vi "Timeout Timer.vi"(1 "reset?(F)":bool, 2 "timeout(s)":dbl=5.0) -> (7 "timeout?":bool, 9 "time esliped?":dbl)   [LabVIEW 2017]
doc: "Reports whether the configured timeout has elapsed and returns the time since the timer was last reset."
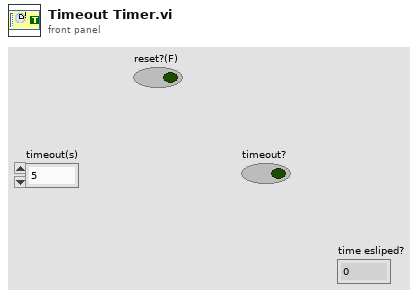
[diagram p1: front panel]
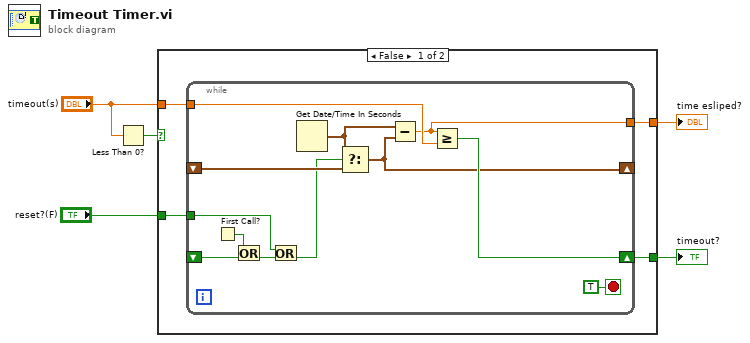
[diagram p0: block diagram]
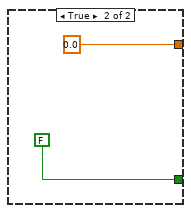
[diagram p2: hidden frame]
diagram:
  n1 = Less Than 0?(x="timeout(s)") -> (x < 0?=w4:bool)
  n2 = case shown="False" w4 {
    tunnel: "timeout(s)" -> [w9 _]
    tunnel: [w8 FALSE] -> w5
    tunnel: [w7 0.0] -> w2
    tunnel: "reset?(F)" -> [w6 _]
    frame False {
      n3 = while {
        shift-right: [w15] -> _
        shift-left: _ -> [w20]
        tunnel: w9 -> [w19]
        shift-right: [w18] -> w8
        shift-left: _ -> [w14]
        tunnel: [w17] -> w7
        tunnel: w6 -> [w10]
        stop <- TRUE stop-if-true
        n4 = First Call?() -> (First Call?: T/F=w12:bool)
        n5 = Or(x=w12, y=w14) -> (x .or. y?=w13:bool)
        n6 = Or(x=w10, y=w13) -> (x .or. y?=w11:bool)
        n7 = Get Date/Time In Seconds() -> (seconds since 1Jan1904=w16:timestamp)
        n8 = Select(t=w16, s=w11, f=w20) -> (s? t:f=w15:timestamp)
        n9 = Subtract(x=w16, y=w15) -> (x-y=w17:dbl)
        n10 = Greater Or Equal?(x=w17, y=w19) -> (x >= y?=w18:bool)
      }
    }
    frame True {
    }
  }
  "timeout?" <- w5
  "time esliped?" <- w2
